vi "Subvi sample and count U8.vi"(6 "Reset":bool, 8 "Clock":bool, 9 "Input":bool) -> (1 "Count":u8)   [LabVIEW 2017]
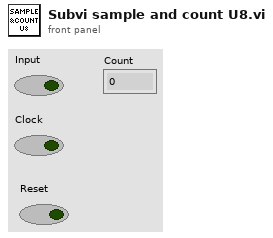
[diagram p1: front panel]
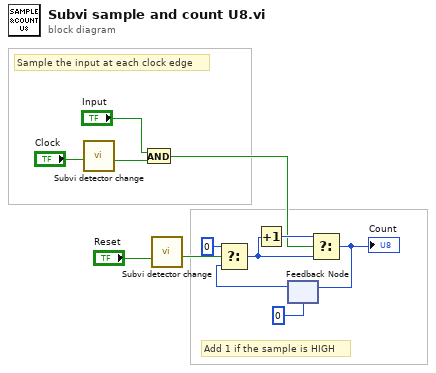
[diagram p0: block diagram]
diagram:
  # "Add 1 if the sample is HIGH"
  # "Sample the input at each clock edge"
  n1 = call "Subvi detector change.vi"("Input"="Clock") -> ("Output"=w4:bool)  [unwired: 8 in]
  n2 = And(x="Input", y=w4) -> (x .and. y?=w1:bool)
  n3 = call "Subvi detector change.vi"("Input"="Reset") -> ("Output"=w5:bool)  [unwired: 8 in]
  n4 = feedback #1(u8 0) -> (w8:u8)
  n5 = Select(t=u8 0, s=w5, f=w8) -> (s? t:f=w7:u8)
  n6 = Increment(x=w7) -> (x+1=w12:u8)
  n7 = Select(t=w12, s=w1, f=w7) -> (s? t:f=w9:u8)
  "Count" <- w9
  n8 = feedback-in #1(w9) -> ()
